vi "backward_dist_calc.vi"(0 "dt":dbl, 2 "Sodar Past":dbl, 3 "Forward Right":dbl, 4 "Sodar":dbl, 5 "Forward Left Past":dbl, 6 "Forward Left":dbl, 7 "Forward Right Past":dbl) -> (1 "Forward distance":dbl)   [LabVIEW 2015]
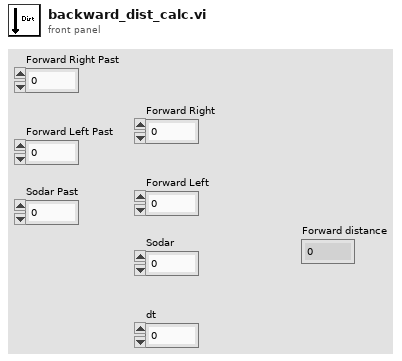
[diagram p1: front panel]
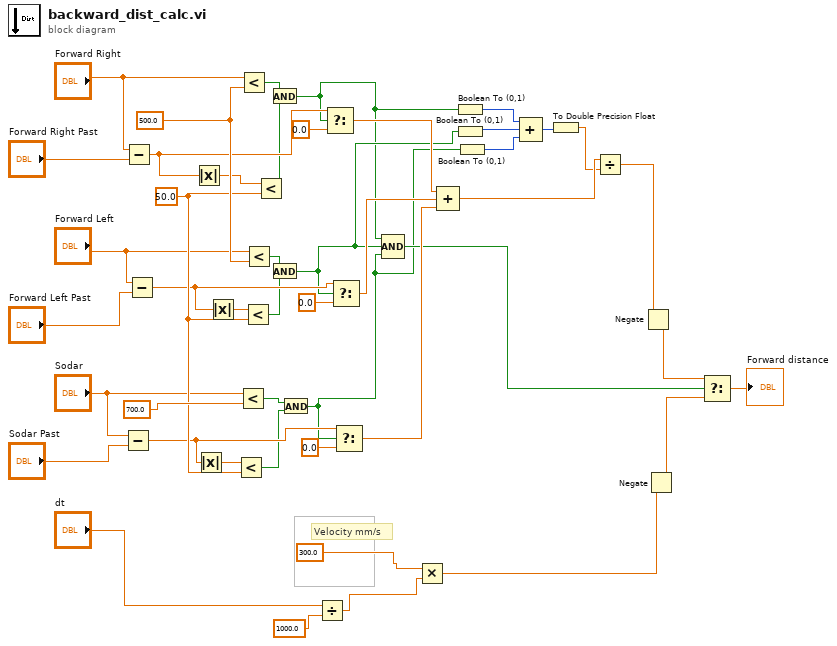
[diagram p0: block diagram]
diagram:
  w22 = 50.0 ("y")
  w46 = 500.0
  # "Velocity mm/s"
  n1 = Subtract(x="Sodar", y="Sodar Past") -> (x-y=w20:dbl)
  n2 = Subtract(x="Forward Right", y="Forward Right Past") -> (x-y=w23:dbl)
  n3 = Subtract(x="Forward Left", y="Forward Left Past") -> (x-y=w21:dbl)
  n4 = Absolute Value(x=w23) -> (abs(x)=w10:dbl)
  n5 = Absolute Value(x=w20) -> (abs(x)=w8:dbl)
  n6 = Absolute Value(x=w21) -> (abs(x)=w9:dbl)
  n7 = Less?(x=w8, y=w22) -> (x < y?=w18:bool)
  n8 = Less?(x="Sodar", y=700.0) -> (x < y?=w19:bool)
  n9 = Less?(x="Forward Right", y=w46) -> (x < y?=w13:bool)
  n10 = Less?(x=w9, y=w22) -> (x < y?=w15:bool)
  n11 = Less?(x="Forward Left", y=w46) -> (x < y?=w16:bool)
  n12 = Less?(x=w10, y=w22) -> (x < y?=w12:bool)
  n13 = And(x=w13, y=w12) -> (x .and. y?=w11:bool)
  n14 = And(x=w16, y=w15) -> (x .and. y?=w14:bool)
  n15 = And(x=w19, y=w18) -> (x .and. y?=w17:bool)
  n16 = Divide(x="dt", y=1000.0) -> (x/y=w24:dbl)
  n17 = Select(t=w23, s=w11, f=0.0) -> (s? t:f=w37:dbl)
  n18 = Select(t=w21, s=w14, f=0.0) -> (s? t:f=w36:dbl)
  n19 = Select(t=w20, s=w17, f=0.0) -> (s? t:f=w35:dbl)
  n20 = Compound Arithmetic op=AND(w11, w14, w17) -> (w28:bool)
  n21 = Multiply(x=300.0, y=w24) -> (x*y=w27:dbl)
  n22 = Compound Arithmetic op=ADD(w37, w36, w35) -> (w30:dbl)
  n23 = Boolean To (0,1)(Boolean=w11) -> (0, 1=w34:i16)
  n24 = Boolean To (0,1)(Boolean=w14) -> (0, 1=w33:i16)
  n25 = Boolean To (0,1)(Boolean=w17) -> (0, 1=w32:i16)
  n26 = Compound Arithmetic op=ADD(w34, w33, w32) -> (w31:i16)
  n27 = To Double Precision Float(number=w31) -> (double precision float=w29:dbl)
  n28 = Divide(x=w30, y=w29) -> (x/y=w4:dbl)
  n29 = Negate(x=w4) -> (-x=w2:dbl)
  n30 = Negate(x=w27) -> (-x=w1:dbl)
  n31 = Select(t=w2, s=w28, f=w1) -> (s? t:f=→"Forward distance":dbl)
